vi "hw2-4 topVI.vi"() -> ()   [LabVIEW 2014]
panel:
  out "Results":dbl[][](array[numeric])
  in  "Num of stairs":i32=5
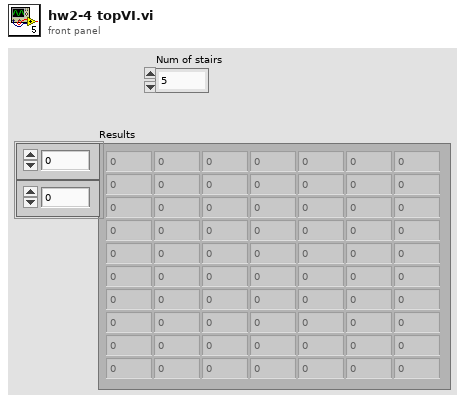
[diagram p1: front panel]
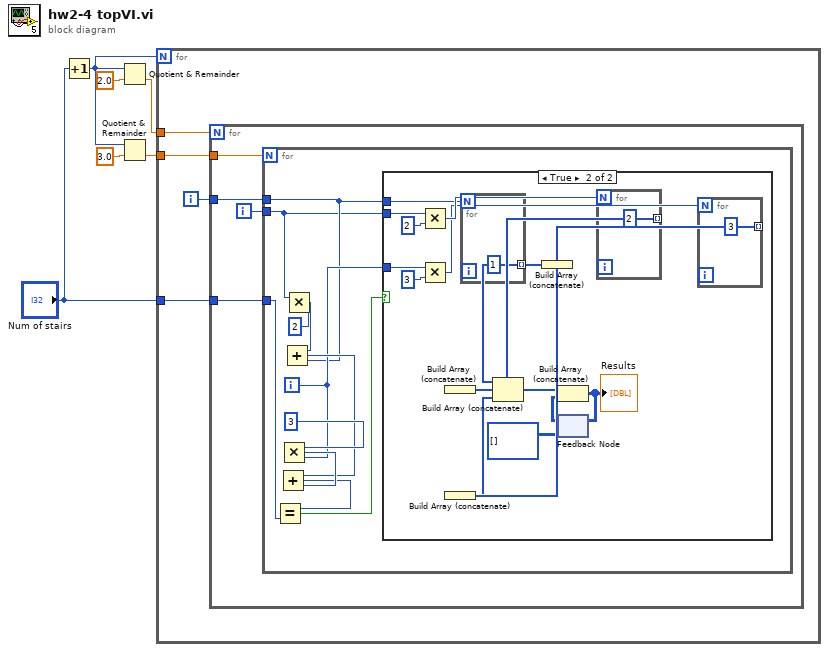
[diagram p0: block diagram]
diagram:
  n1 = Increment(x="Num of stairs") -> (x+1=w2:i32)
  n2 = Quotient & Remainder(x=w2, y=2.0) -> (floor(x/y)=w4:dbl)  [unwired: 1 out]
  n3 = Quotient & Remainder(x=w2, y=3.0 ("x")) -> (floor(x/y)=w3:dbl)  [unwired: 1 out]
  n4 = for {
    N: w2 -> [_]
    tunnel: w4 -> [w10]
    tunnel: w3 -> [w9]
    tunnel: "Num of stairs" -> [w7]
    i -> [w8]
    n5 = for {
      N: w10 -> [_]
      tunnel: w9 -> [w14]
      tunnel: w8 -> [w13]
      tunnel: w7 -> [w11]
      i -> [w12]
      n6 = for {
        N: w14 -> [_]
        tunnel: w13 -> [w17]
        tunnel: w12 -> [w16]
        tunnel: w11 -> [w15]
        i -> [w18]
        n7 = Multiply(x=3, y=w18) -> (x*y=w22:i32)
        n8 = Multiply(x=w16, y=2) -> (x*y=w20:i32)
        n9 = Add(x=w20, y=w17) -> (x+y=w19:i32)
        n10 = Add(x=w19, y=w22) -> (x+y=w21:i32)
        n11 = Equal?(x=w21, y=w15) -> (x = y?=w25:bool)
        n12 = case shown="True" w25 {
          tunnel: w17 -> [_ w30]
          tunnel: w16 -> [_ w32]
          tunnel: w18 -> [_ w31]
          frame False {
          }
          frame True {
            n13 = Multiply(x=w32, y=2) -> (x*y=w36:i32)
            n14 = Multiply(x=w31, y=3) -> (x*y=w34:i32)
            n15 = for {
              N: w30 -> [_]
              tunnel: [1] -> w42 mode=indexing
            }
            n16 = Build Array (concatenate)(w42) -> (w39:i32[])
            n17 = feedback #1(i32[][] []) -> (w27:i32[][])
            n18 = for {
              N: w36 -> [_]
              tunnel: [2] -> w41 mode=indexing
            }
            n19 = Build Array (concatenate)(w41) -> (w38:i32[])
            n20 = for {
              N: w34 -> [_]
              tunnel: [3] -> w40 mode=indexing
            }
            n21 = Build Array (concatenate)(w40) -> (w37:i32[])
            n22 = Build Array (concatenate)(w39, w38, w37) -> (w29:i32[])
            n23 = Build Array (concatenate)(w29, w27) -> (w28:i32[][])
            "Results" <- w28
            n24 = feedback-in #1(w28) -> ()
          }
        }
      }
    }
  }
